vi "S8300E_WritetMAC.vi"() -> ()   [LabVIEW 2011]
panel:
  out "PORT1_MAC":string
  out "UUT MAC List":string
  out "CMD-LIST":cluster{string, string, string, string}[](array[cluster])
  out "log msg":string
  out "VISA resource name out":refnum<visa-resource-name>
  out "BEGIN TIME":u32
  out "進行狀況":string
  # "Error Code:MAC-PORT1\nError Code:MAC-PORT2\nError Code:MAC-PORT3"
  # "2014-12-15"
  # "S8300E UUT 3 Ports MAC (接UART COM9)"
  # "Write 3 Ports  MAC Address"
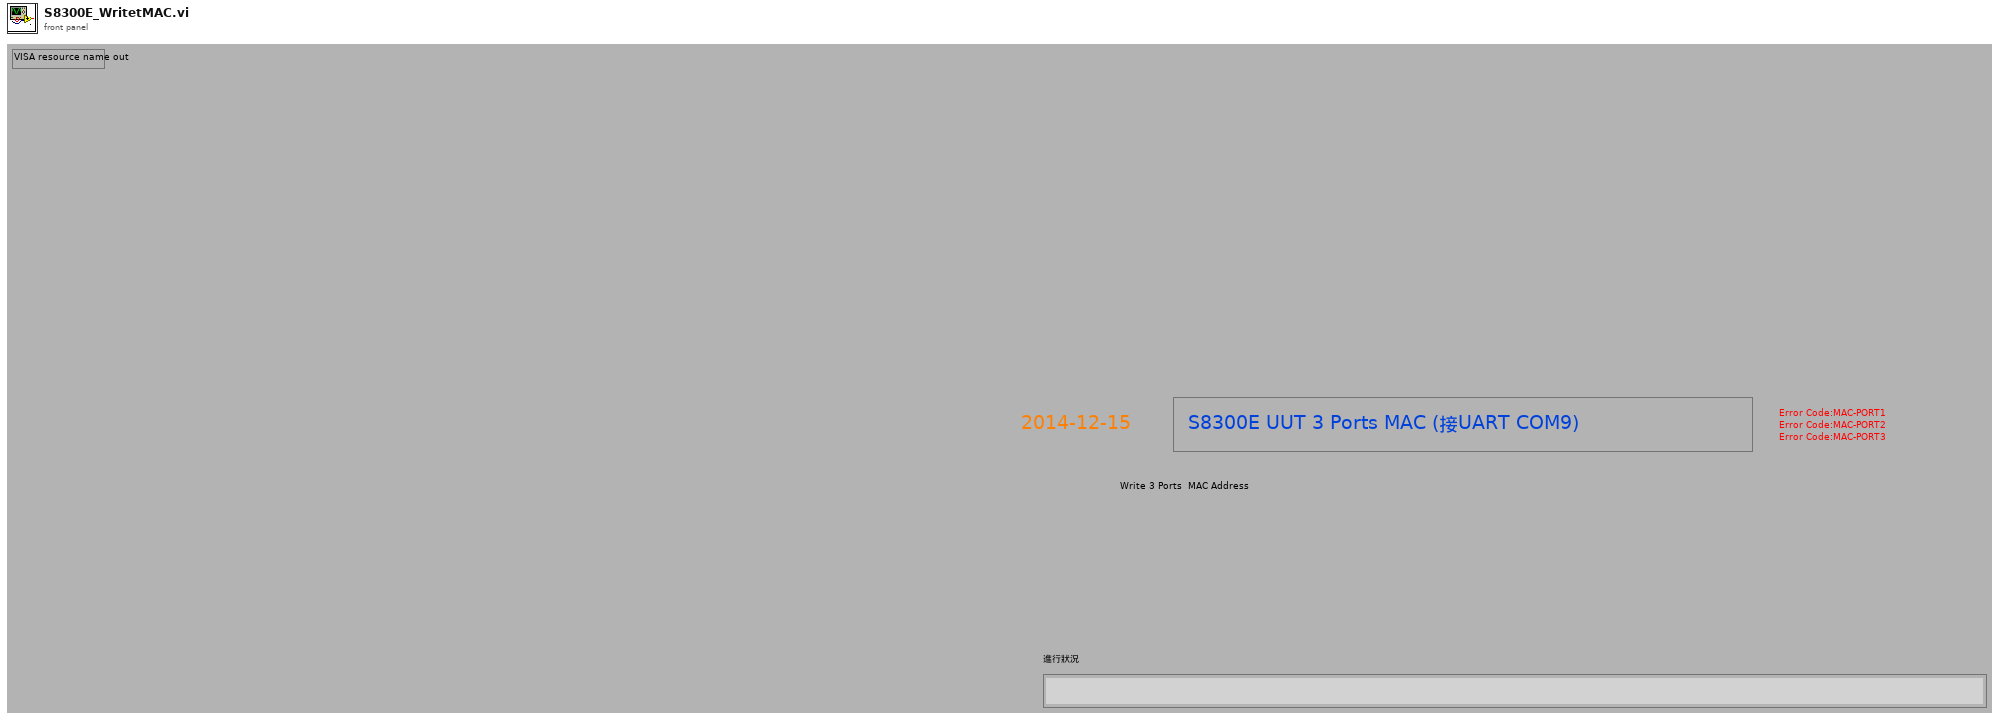
[diagram p1: front panel]
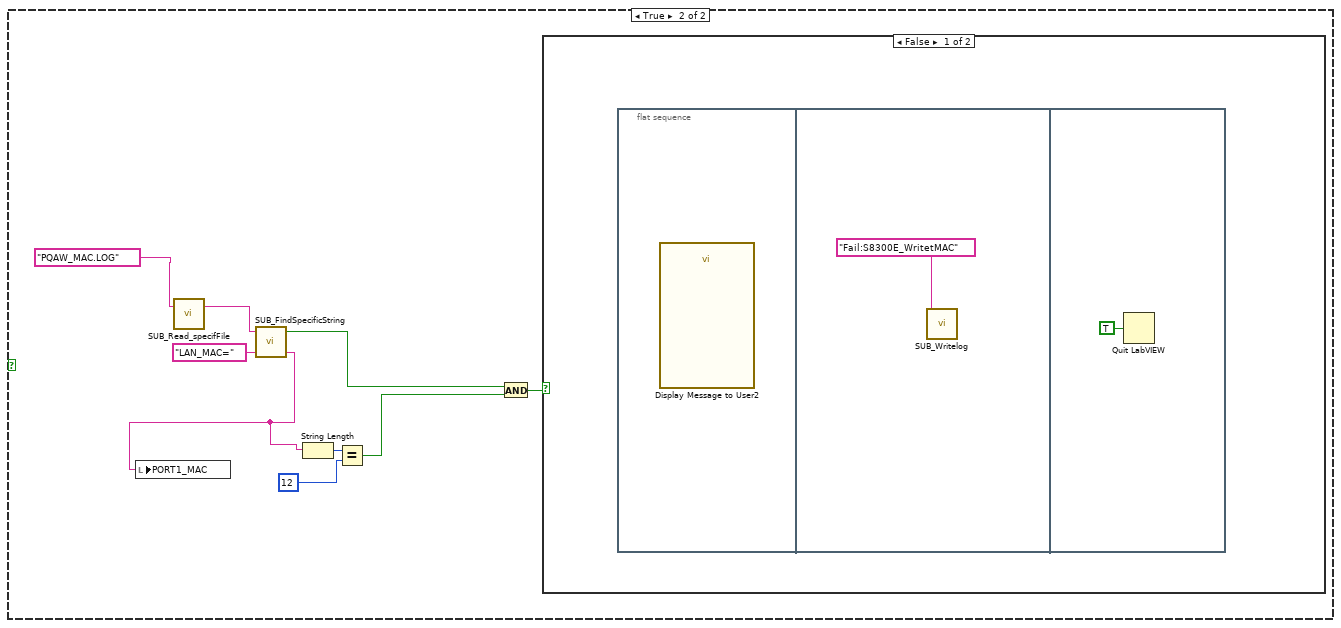
[diagram p3: hidden frame]
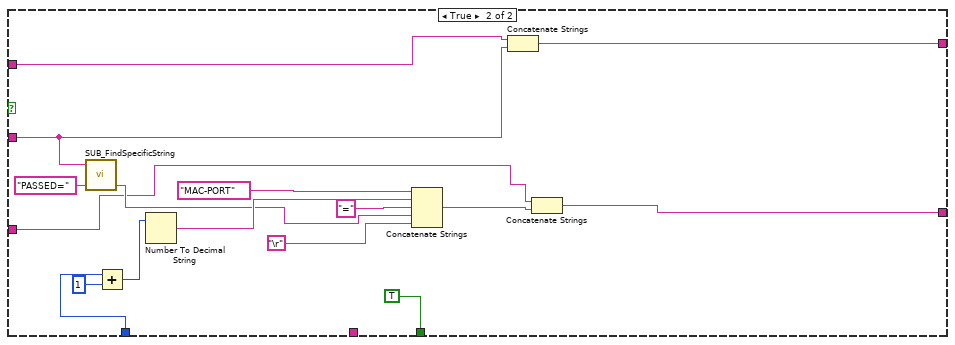
[diagram p7: hidden frame]
diagram:
  n1 = flat-sequence {
    frame #0 {
      n2 = Tick Count (ms)() -> (millisecond timer value=→"BEGIN TIME":u32)
    }
    frame #1 {
      n3 = property on="進行狀況" class="Str"("Blinking"=TRUE) -> ()  [unwired: 2 in, 2 out]
      "進行狀況" <- "進入測試準備中...." ("進行狀況")
      "PORT1_MAC" <- ""
    }
    frame #2 {
      n4 = call "SUB_SearchFile_inFolder.vi"("Search Filename in Folder"="S8300E_sfcs_misc.txt") -> ("File Existing True/Flase"=w5:bool)  [unwired: 1 in]
      n5 = case shown="False" w5 {
        frame False {
          n6 = flat-sequence {
            frame #0 {
              n7 = call "Display Message to User"() -> ()  [unwired: 10 in, 2 out]
            }
            frame #1 {
              n8 = call "SUB_Writelog.vi"("Pass/Fail"="Fail:S8300E_WritetMAC") -> ()  [unwired: 2 in]
            }
            frame #2 {
              n9 = Quit LabVIEW(quit? (T)=TRUE) -> ()
            }
          }
        }
        frame True {
        }
      }
    }
    frame #3 {
    }
    frame #4 {
      n10 = call "SUB_SearchFile_inFolder.vi"("Search Filename in Folder"="PQAW_MAC.LOG") -> ("File Existing True/Flase"=w9:bool)  [unwired: 1 in]
      n11 = case shown="False" w9 {
        frame False {
          n12 = flat-sequence {
            frame #0 {
              n13 = call "Display Message to User3"() -> ()  [unwired: 10 in, 2 out]
            }
            frame #1 {
              n14 = call "SUB_Writelog.vi"("Pass/Fail"="Fail:S8300E_WritetMAC") -> ()  [unwired: 2 in]
            }
            frame #2 {
              n15 = Quit LabVIEW(quit? (T)=TRUE) -> ()
            }
          }
        }
        frame True {
          n16 = call "SUB_Read_specifFile.vi"("name or relative path"="PQAW_MAC.LOG" ("Search Filename in Folder")) -> ("text"=w20:string)  [unwired: 1 in, 1 out]
          n17 = call "SUB_FindSpecificString.vi"("Find this String"="LAN_MAC=", "String data"=w20) -> ("before \"; \" string"=w18:string, "Found"=w14:bool)  [unwired: 2 in]
          n18 = local write "PORT1_MAC"(w18) -> ()
          n19 = String Length(string=w18) -> (length=w17:i32)
          n20 = Equal?(x=w17, y=12) -> (x = y?=w13:bool)
          n21 = And(x=w14, y=w13) -> (x .and. y?=w15:bool)
          n22 = case shown="False" w15 {
            frame False {
              n23 = flat-sequence {
                frame #0 {
                  n24 = call "Display Message to User2"() -> ()  [unwired: 10 in, 2 out]
                }
                frame #1 {
                  n25 = call "SUB_Writelog.vi"("Pass/Fail"="Fail:S8300E_WritetMAC") -> ()  [unwired: 2 in]
                }
                frame #2 {
                  n26 = Quit LabVIEW(quit? (T)=TRUE) -> ()
                }
              }
            }
            frame True {
            }
          }
        }
      }
    }
    frame #5 {
      n27 = local read "PORT1_MAC"() -> (w30:string)
      n28 = call "SUB_Gen3ports_MACString.vi"("Port1-MAC Input"=w30) -> ("port3-MAC"=w24:string, "port2-MAC"=w27:string, "port1-MAC"=w28:string)  [unwired: 2 in]
      n29 = Concatenate Strings("./mac.sh -w -e  1  ", w28, "\r") -> (w48:string)
      n30 = Concatenate Strings("./mac.sh -w -e  2  ", w27, "\r") -> (w44:string)
      n31 = Concatenate Strings("./mac.sh -w -e  3 ", w24, "\r") -> (w40:string)
      n32 = Bundle(w48, "PASSED=", "Programming  MAC-PORT1..", "MAC-PORT1") -> (w34:cluster{string, string, string, string})  [unwired: 1 in]
      n33 = Bundle(w44, "PASSED=", "Programming   MAC-PORT2...", "MAC-PORT2") -> (w33:cluster{string, string, string, string})  [unwired: 1 in]
      n34 = Bundle(w40, "PASSED=", "Programming  MAC-PORT3...", "MAC-PORT3") -> (w32:cluster{string, string, string, string})  [unwired: 1 in]
      n35 = Build Array(w34, w33, w32) -> (→"CMD-LIST":cluster{string, string, string, string}[])
    }
    frame #6 {
      n36 = call "SUB_COM1_CLOSE.vi"("VISA resource name"=refnum<visa-resource-name> "COM9") -> ()  [unwired: 3 in]
    }
    frame #7 {
      n37 = case shown="True" TRUE {
        frame False {
        }
        frame True {
          n38 = call "SUB_COM9_INIT.vi"("baud rate"=u32 115200) -> ("VISA resource name out"=w55:refnum<visa-resource-name>)  [unwired: 1 in, 1 out]
          "VISA resource name out" <- w55
          n39 = call "SUB_COM1Wrt.vi"("VISA resource name"=w55, "write buffer"="\r") -> ("duplicate VISA resource name"=w52:refnum<visa-resource-name>)  [unwired: 1 in, 1 out]
          n40 = call "SUB_ContinueCom1Read.vi"("Numeric"=3600, "duplicate VISA resource name 2"=w52) -> ()  [unwired: 1 in, 3 out]
        }
      }
    }
    frame #8 {
      n41 = local read "CMD-LIST"() -> (w59:cluster{string, string, string, string}[])
      n42 = Array Size(array=w59) -> (size(s)=w62:i32)
      n43 = for {
        N: w62 -> [_]
        shift-right: [w67] -> w60
        shift-left: "" -> [w66]
        shift-right: [w64] -> w57
        shift-left: "" -> [w63]
        i -> [w65]
        n44 = while {
          tunnel: w65 -> [w86]
          tunnel: [w78] -> w67
          tunnel: w66 -> [w77]
          tunnel: w65 -> [w70]
          tunnel: [w69] -> w64
          tunnel: w63 -> [w68]
          stop <- w80 stop-if-true
          n45 = local read "VISA resource name out"() -> (w82:refnum<visa-resource-name>)
          n46 = local read "CMD-LIST"() -> (w76:cluster{string, string, string, string}[])
          n47 = Index Array(array=w76, index=w86) -> (element=w75:cluster{string, string, string, string})
          n48 = Unbundle(w75) -> (w74:string, w72:string, w73:string, w71:string)
          n49 = call "SUB_COM1Wrt.vi"("VISA resource name"=w82, "write buffer"=w74) -> ("duplicate VISA resource name"=w85:refnum<visa-resource-name>)  [unwired: 1 in, 1 out]
          n50 = Tick Count (ms)() -> (millisecond timer value=w84:u32)
          n51 = call "SUB_READ_COM1_FindString_timeout.vi"("Find this String"=w72, "Timeout Seccond"=5.0, "Begin time"=w84, "duplicate VISA resource name 2"=w85) -> ("Output String"=w79:string, "Found String"=w81:bool)  [unwired: 1 in, 1 out]
          n52 = local write "進行狀況"(w73) -> ()
          n53 = case shown="False" w81 {
            tunnel: [_ TRUE] -> w80
            tunnel: w79 -> [w97 w114]
            tunnel: [w93 w119] -> w78
            tunnel: w77 -> [w93 w118]
            tunnel: w71 -> [w92 _]
            tunnel: w70 -> [_ w110]
            tunnel: [w87 w106] -> w69
            tunnel: w68 -> [w87 w105]
            frame False {
              n54 = local read "進行狀況"() -> (w89:string)
              n55 = Concatenate Strings("寫錄MAC失敗!" ("string"), "\r", w89) -> (w88:string)
              n56 = call "SUB_YESNO.vi"("Debug View"=w97, "Status"=w88) -> ("yes/no"=w96:enum32{"No Selection", "Yes", "No", "None"})  [unwired: 1 in]
              n57 = Equal?(x=w96, y=enum32{"No Selection", "Yes", "No", "None"}."No") -> (x = y?=w94:bool)
              n58 = case shown="True" w94 {
                tunnel: w92 -> [_ w98]
                frame False {
                }
                frame True {
                  n59 = flat-sequence {
                    tunnel: [w100] -> w99
                    tunnel: w98 -> [w100]
                    tunnel: w99 -> [w102]
                    frame #0 {
                      n60 = call "SUB_Writelog.vi"("Pass/Fail"="Fail:S8300E_WritetMAC") -> ()  [unwired: 2 in]
                    }
                    frame #1 {
                      n61 = call "SUB_SFCS_SendResult.vi"("ErrorCode"=w102, "PASS_Fail (1/0)"=i8 0) -> ()  [unwired: 1 out]
                    }
                    frame #2 {
                      n62 = Quit LabVIEW(quit? (T)=TRUE) -> ()
                    }
                  }
                }
              }
            }
            frame True {
              n63 = call "SUB_FindSpecificString.vi"("Find this String"="PASSED=", "String data"=w114) -> ("before \"; \" string"=w112:string)  [unwired: 2 in, 1 out]
              n64 = Add(x=w110, y=1) -> (x+y=w108:i32)
              n65 = Number To Decimal String(number=w108) -> (decimal integer string=w116:string)  [unwired: 1 in]
              n66 = Concatenate Strings("MAC-PORT" ("string"), w116, "=" ("string"), w112, "\r") -> (w107:string)
              n67 = Concatenate Strings(w118, w114) -> (w119:string)
              n68 = Concatenate Strings(w105, w107) -> (w106:string)
            }
          }
        }
      }
      "log msg" <- w60
      "UUT MAC List" <- w57
    }
    frame #9 {
      n69 = call "SUB_COM1_CLOSE.vi"("VISA resource name"=refnum<visa-resource-name> "COM9") -> ()  [unwired: 3 in]
    }
    frame #10 {
      n70 = local read "log msg"() -> (w122:string)
      n71 = local read "BEGIN TIME"() -> (w128:u32)
      n72 = Tick Count (ms)() -> (millisecond timer value=w127:u32)
      n73 = call "SUB_CAL_TESTTIME.vi"("Test Item name"="S8300E_WritetMAC", "Stop tick time"=w127, "Start tick time"=w128) -> ("Test Time output"=w124:string)  [unwired: 2 in]
      n74 = Concatenate Strings("Pass:S8300E_WritetMAC", "\n", w122, w124) -> (w125:string)
      n75 = call "SUB_Writelog.vi"("Pass/Fail"=w125) -> ()  [unwired: 2 in]
    }
    frame #11 {
      n76 = Request Deallocation(TRUE ("flag")) -> ()
    }
    frame #12 {
      n77 = Quit LabVIEW(quit? (T)=TRUE ("stop? (T)")) -> ()
    }
  }
